vi "Auto-Search.vi"(2 "Counter\\Timer":dbl, 3 "Low Angle Edge":dbl, 4 "High Angle Edge":dbl) -> (0 "counter":dbl, 1 "Servo Angle":dbl)   [LabVIEW 2011]
panel:
  out "s? t:f":dbl(knob) scale=0.0..200.0
  out "Angle":dbl
  out "R":dbl
  in  "Last Angle":dbl
  in  "Low Angle Edge":dbl
  in  "High Angle Edge":dbl
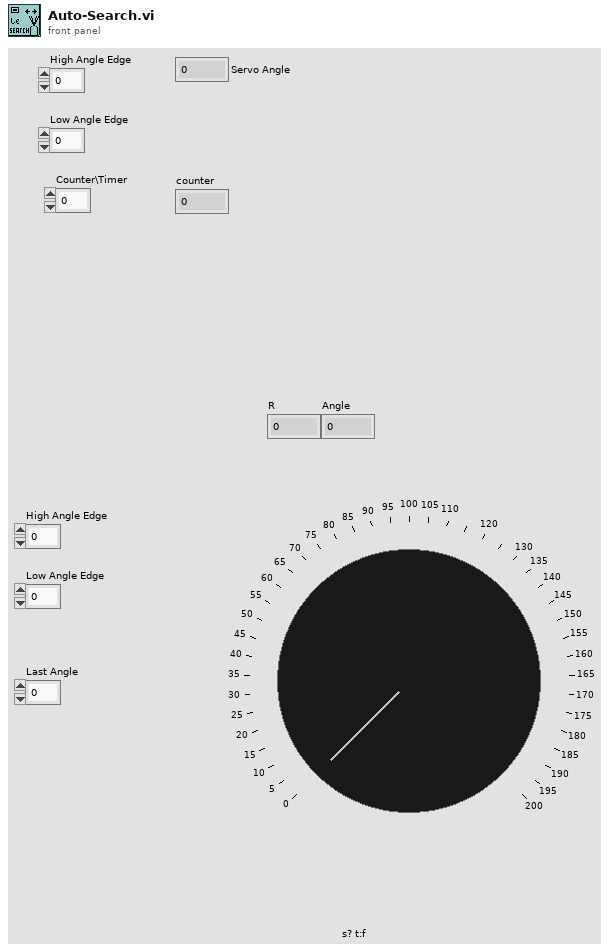
[diagram p1: front panel]
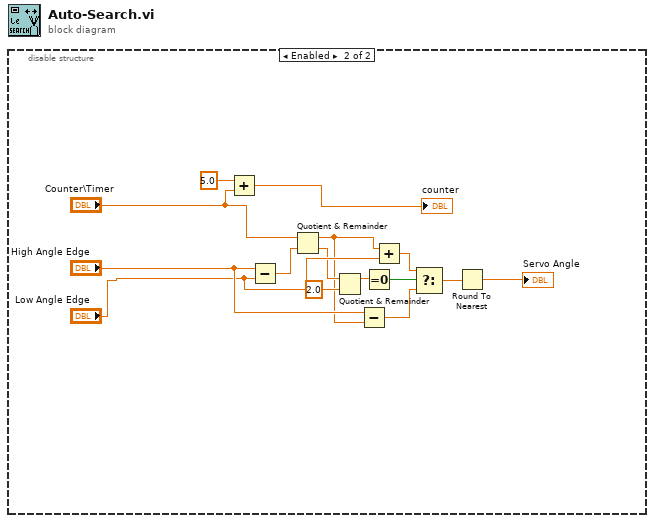
[diagram p0: block diagram]
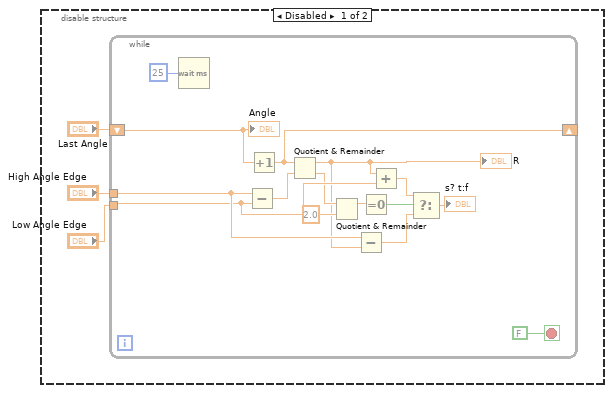
[diagram p2: hidden frame]
diagram:
  n1 = disable-structure shown="Enabled" {
    frame Disabled {
      n2 = while {
        tunnel: "Low Angle Edge" -> [w13]
        tunnel: "High Angle Edge" -> [w14]
        shift-right: [w16] -> _
        shift-left: "Last Angle" -> [w18]
        stop <- FALSE stop-if-true
        n3 = Wait (ms)(milliseconds to wait=u32 25) -> ()  [unwired: 1 out]
        n4 = Subtract(x=w14, y=w13) -> (x-y=w12:dbl)
        n5 = Increment(x=w18) -> (x+1=w16:dbl)
        n6 = Quotient & Remainder(x=w16, y=w12) -> (x-y*floor(x/y)=w5:dbl, floor(x/y)=w11:dbl)
        "R" <- w5
        n7 = Quotient & Remainder(x=w11, y=2.0) -> (x-y*floor(x/y)=w9:dbl)  [unwired: 1 out]
        n8 = Subtract(x=w14, y=w5) -> (x-y=w7:dbl)
        n9 = Equal To 0?(x=w9) -> (x = 0?=w8:bool)
        n10 = Add(x=w5, y=w13) -> (x+y=w4:dbl)
        n11 = Select(t=w4, s=w8, f=w7) -> (s? t:f=→"s? t:f":dbl)
        "Angle" <- w18
      }
    }
    frame Enabled {
      n12 = Add(x=5.0, y="Counter\\Timer") -> (x+y=→"counter":dbl)
      n13 = Subtract(x="High Angle Edge", y="Low Angle Edge") -> (x-y=w31:dbl)
      n14 = Quotient & Remainder(x="Counter\\Timer", y=w31) -> (x-y*floor(x/y)=w25:dbl, floor(x/y)=w30:dbl)
      n15 = Quotient & Remainder(x=w30, y=2.0) -> (x-y*floor(x/y)=w28:dbl)  [unwired: 1 out]
      n16 = Subtract(x="High Angle Edge", y=w25) -> (x-y=w26:dbl)
      n17 = Equal To 0?(x=w28) -> (x = 0?=w27:bool)
      n18 = Add(x=w25, y="Low Angle Edge") -> (x+y=w24:dbl)
      n19 = Select(t=w24, s=w27, f=w26) -> (s? t:f=w23:dbl)
      n20 = Round To Nearest(number=w23) -> (nearest integer value=→"Servo Angle":dbl)
    }
  }
